vi "CMI Sync V3 Panel.vi"(8 "error in":errorcluster, 11 "session in":T2={"VISA"="", "baud rate [bd/s]"=115200, "source"=enum."Auto", "hv range"=enum."1kV", "fsrc is fixed"=FALSE, "fsrc [Hz]"=10000000.0, "freq integ [s]"=1.0, "freq filter"=5, "trig level"=enum."TTL 5V", "chn1 mode"=enum."Source divider", "chn1 level"=enum."Positive 5V", "chn2 mode"=enum."Source divider", "chn2 level"=enum."Positive 5V", "chn2 div"=1, "chn3 mode"=enum."Chn 1 Active", "chn3 level"=enum."Positive 5V", "chn1 div entry"=enum."Calculate nearest divisor from measured fx", "chn1 dev limit [%]"=1.0, "chn1 check dev"=FALSE} {"chn2 div" min=1 max=100000000 step=1; "fsrc [Hz]" format="%_8p"}) -> (0 "error out":errorcluster, 3 "session out":T2={"VISA"="", "baud rate [bd/s]"=115200, "source"=enum."Auto", "hv range"=enum."1kV", "fsrc is fixed"=FALSE, "fsrc [Hz]"=10000000.0, "freq integ [s]"=1.0, "freq filter"=5, "trig level"=enum."TTL 5V", "chn1 mode"=enum."Source divider", "chn1 level"=enum."Positive 5V", "chn2 mode"=enum."Source divider", "chn2 level"=enum."Positive 5V", "chn2 div"=1, "chn3 mode"=enum."Chn 1 Active", "chn3 level"=enum."Positive 5V", "chn1 div entry"=enum."Calculate nearest divisor from measured fx", "chn1 dev limit [%]"=1.0, "chn1 check dev"=FALSE} {"chn2 div" min=1 max=100000000 step=1; "fsrc [Hz]" format="%_8p"})   [LabVIEW 2020, in "AWG.lvlib" / "CMI Sync Unit V3.lvlib"]
doc: "Configuration panel of CMI Sync Unit V3. Sets the basic setup that is not intended to be changed after opening the device."
uses:
  CMI Sync Unit V3.lvlib
  varilib/varilib.lvlib
  varilib/SGUI Assign References Mode.ctl
  varilib/SGUI Assign Multiple Strings With Tags By Label.vi
  Configure/CMI Sync V3 Reference Clock Source.ctl
  Configure/CMI Sync V3 Channel 1 Mode.ctl
  Configure/CMI Sync V3 Channel 1 Divisor Entry Mode.ctl
  varilib/SGUI Set Single Real By Label.vi
  Configure/CMI Sync V3 HV input Range.ctl
  Configure/CMI Sync V3 Trigger Input Level.ctl
  Configure/CMI Sync V3 Channel 2 Mode.ctl
  Configure/CMI Sync V3 Channel Output Levels.ctl
  Configure/CMI Sync V3 Channel 3 Mode.ctl
  CMI Sync V3 session.ctl
panel:
  in  "chn1 freq limit":dbl=0.01 caption="Freq limit [%]" min=1e-09 max=100.0 step=0.01
  in  "chn1 check limit":bool caption="Channel 1 check deviation limit"
  in  "chn1 div entry":T1=enum."Calculate nearest divisor from measured fx" caption="Channel 1 source divider mode"
  out "err string":string caption="Error"
  out "meas freq":dbl caption="Source frequency [Hz]" format="%0_8p"
  out "idn string":string caption="Device identification"
  in  "btn check":bool
  in  "btn ok":bool caption="OK"
  in  "fsrc":dbl=10000000.0 caption="Source frequency [Hz]" format="%_8p"
  in  "fsrc fixed":bool caption="Define source freq. here:"
  in  "chn3 level":T7=enum."Positive 5V" caption="Channel 3 output levels"
  in  "chn3 mode":T9 caption="Channel 3 mode"
  in  "chn2 level":T7=enum."Positive 5V" caption="Channel 2 output levels"
  in  "chn1 level":T7=enum."Positive 5V" caption="Channel 1 output levels"
  in  "chn2 div":i32=1 caption="Channel 2 divisor" min=1 max=100000000 step=1
  in  "chn2 mode":T8 caption="Channel 2 mode"
  in  "trig level":T5=enum."TTL 5V" caption="Trigger input logic"
  in  "freq filter":i32=5 caption="Counter filtering periods"
  in  "freq integ":dbl=1.0 caption="Counter integration [s]"
  in  "chn1 mode":T6 caption="Channel 1 mode"
  in  "hv range":T4=enum."1kV" caption="HV input range"
  in  "VISA address":refnum<visa-resource-name>
  in  "source":T3 caption="Clock source"
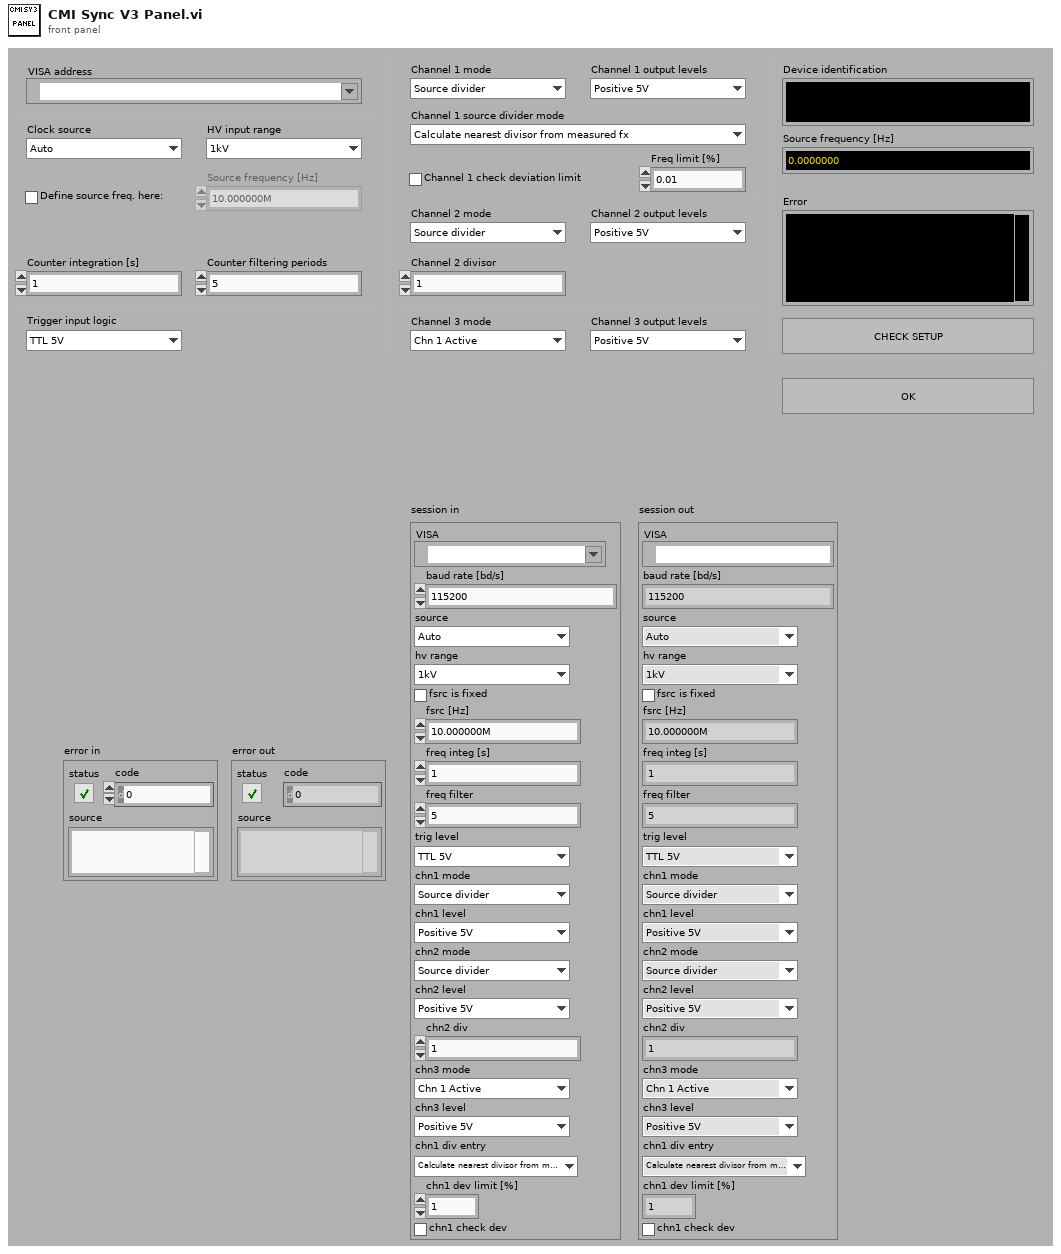
[diagram p1: front panel]
types:
  T1 = typedef "AWG.lvlib/CMI Sync Unit V3.lvlib/CMI Sync V3 Channel 1 Divisor Entry Mode.ctl" = enum16{"Set divisor directly", "Calculate nearest divisor from measured fx"}
  T2 = typedef "AWG.lvlib/CMI Sync Unit V3.lvlib/CMI Sync V3 session.ctl" = cluster{"VISA":refnum<visa-resource-name>, "baud rate [bd/s]":i32, "source":T3, "hv range":T4, "fsrc is fixed":bool, "fsrc [Hz]":dbl, "freq integ [s]":dbl, "freq filter":i32, "trig level":T5, "chn1 mode":T6, "chn1 level":T7, "chn2 mode":T8, "chn2 level":T7, "chn2 div":i32, "chn3 mode":T9, "chn3 level":T7, "chn1 div entry":T1, "chn1 dev limit [%]":dbl, "chn1 check dev":bool}
  T3 = typedef "AWG.lvlib/CMI Sync Unit V3.lvlib/CMI Sync V3 Reference Clock Source.ctl" = enum16{"Auto", "Internal", "Logic", "Sine", "HV"}
  T4 = typedef "AWG.lvlib/CMI Sync Unit V3.lvlib/CMI Sync V3 HV input Range.ctl" = enum16{"10V", "60V", "250V", "1kV"}
  T5 = typedef "AWG.lvlib/CMI Sync Unit V3.lvlib/CMI Sync V3 Trigger Input Level.ctl" = enum16{"LVCMOS 3V3", "TTL 5V"}
  T6 = typedef "AWG.lvlib/CMI Sync Unit V3.lvlib/CMI Sync V3 Channel 1 Mode.ctl" = enum16{"Source divider", "DDS absolute", "DDS ratio", "DDS ratio M/N"}
  T7 = typedef "AWG.lvlib/CMI Sync Unit V3.lvlib/CMI Sync V3 Channel Output Levels.ctl" = enum16{"Positive 3V3", "Negative 3V3", "Positive 5V", "Negative 5V"}
  T8 = typedef "AWG.lvlib/CMI Sync Unit V3.lvlib/CMI Sync V3 Channel 2 Mode.ctl" = enum16{"Source divider", "Chn 1 divide"}
  T9 = typedef "AWG.lvlib/CMI Sync Unit V3.lvlib/CMI Sync V3 Channel 3 Mode.ctl" = enum16{"Chn 1 Active", "Chn 2 Active", "Chn 1 Trigger", "Chn 2 Trigger", "Gate", "PPS", "10MHz"}
  T10 = typedef "varilib.lvlib/SGUI Assign References Mode.ctl" = enum16{"Add to stack", "Overwrite", "Release last", "Release ID"}
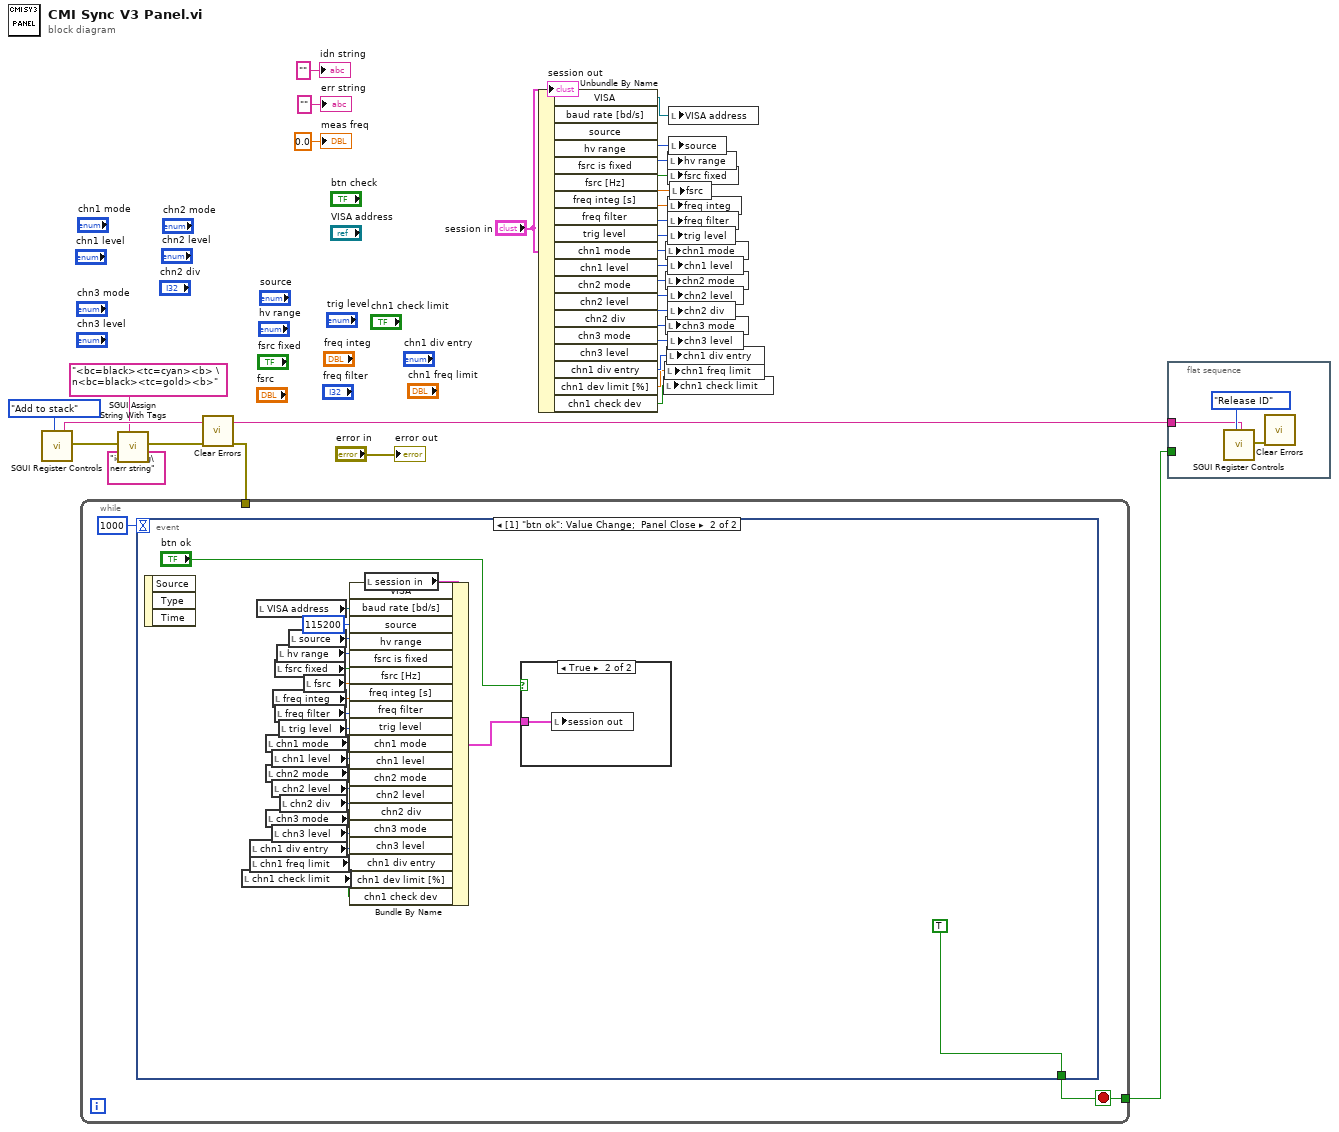
[diagram p0: block diagram]
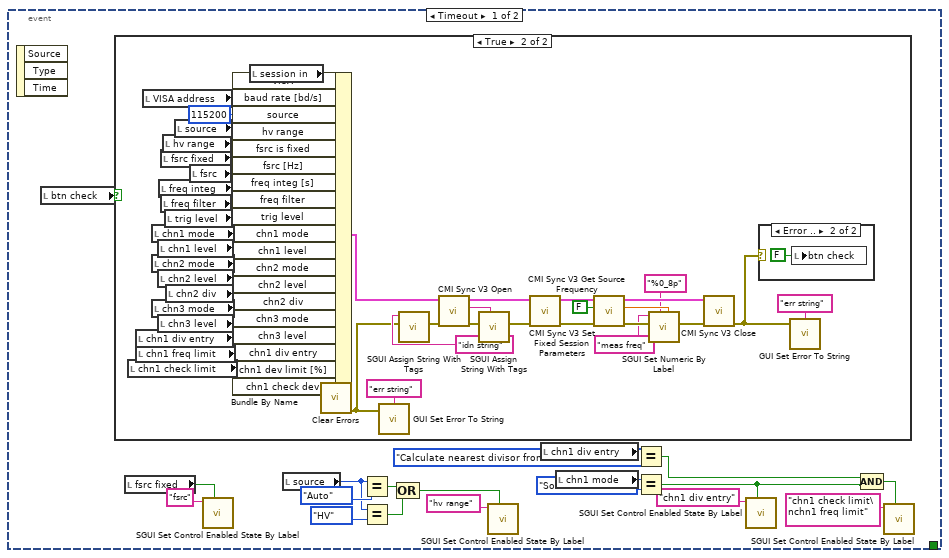
[diagram p2: hidden frame]
diagram:
  n1 = call "SGUI Register Controls.vi"("register mode (overwrite)"=SGUI_Assign_References_Mode."Add to stack") -> ("assigned ID"=w27:string, "error out"=w24:errorcluster)  [unwired: 16 in, 1 out]
  n2 = call-poly "SGUI Assign String With Tags.vi"("error in"=w24, "label(s) (empty)"="idn string\nerr string" ("control label (none)"), "string (empty)"="<bc=black><tc=cyan><b> \n<bc=black><tc=gold><b>" ("control label (none)")) -> ("error out"=w23:errorcluster)  [unwired: 7 in, 1 out]
  n3 = call <vilib>:"Clear Errors.vi"("error in (no error)"=w23) -> ("error out"=w25:errorcluster)  [unwired: 5 in, 1 out]
  n4 = while {
    tunnel: [w33] -> w26
    tunnel: w25 -> [_]
    stop <- w33 stop-if-true
    n5 = event shown="[1] \"btn ok\": Value Change;  Panel Close" {
      selector: _ -> [_ _]
      dyn-events: _ -> [_ _]
      timeout: 1000 -> [_ _]
      tunnel: [_ TRUE] -> w33
      event Timeout {
        n6 = event-data() -> ()  [unwired: 1 in, 3 out]
        n7 = local read "btn check"() -> (w52:bool)
        n8 = case shown="True" w52 {
          frame False {
          }
          frame True {
            w58 = "idn string" ("control label (none)")
            n9 = local read "chn1 check limit"() -> (w53:bool)
            n10 = local read "chn1 div entry"() -> (w55:T1)
            n11 = local read "chn1 freq limit"() -> (w54:dbl)
            n12 = local read "VISA address"() -> (w92:refnum<visa-resource-name>)
            n13 = local read "chn1 mode"() -> (w84:T6)
            n14 = local read "chn2 mode"() -> (w82:T8)
            n15 = local read "chn3 mode"() -> (w79:T9)
            n16 = local read "chn1 level"() -> (w83:T7)
            n17 = local read "chn2 level"() -> (w81:T7)
            n18 = local read "chn3 level"() -> (w78:T7)
            n19 = local read "freq integ"() -> (w87:dbl)
            n20 = local read "fsrc fixed"() -> (w89:bool)
            n21 = local read "freq filter"() -> (w86:i32)
            n22 = local read "hv range"() -> (w90:T4)
            n23 = local read "trig level"() -> (w85:T5)
            n24 = local read "chn2 div"() -> (w80:i32)
            n25 = local read "source"() -> (w91:T3)
            n26 = local read "fsrc"() -> (w88:dbl)
            n27 = local read "session in"() -> (w60:T2)
            n28 = Bundle By Name(cluster=w60, "VISA"=w92, "baud rate [bd/s]"=115200, "source"=w91, "hv range"=w90, "fsrc is fixed"=w89, "fsrc [Hz]"=w88, "freq integ [s]"=w87, "freq filter"=w86, "trig level"=w85, "chn1 mode"=w84, "chn1 level"=w83, "chn2 mode"=w82, "chn2 level"=w81, "chn2 div"=w80, "chn3 mode"=w79, "chn3 level"=w78, "chn1 div entry"=w55, "chn1 dev limit [%]"=w54, "chn1 check dev"=w53) -> (w76:T2)
            n29 = call <vilib>:"Clear Errors.vi"() -> ("error out"=w56:errorcluster)  [unwired: 6 in, 1 out]
            n30 = call "GUI Set Error To String.vi"("error in (no error)"=w56, "label(s) (status)"="err string") -> ()  [unwired: 3 in]
            n31 = call-poly "SGUI Assign String With Tags.vi"("error in"=w56, "label(s) (empty)"=w58) -> ("error out"=w59:errorcluster)  [unwired: 8 in, 1 out]
            n32 = call "CMI Sync V3 Open.vi"("error in"=w59, "session in"=w76) -> ("error out"=w69:errorcluster, "identification string"=w67:string, "session out"=w75:T2)  [unwired: 7 in]
            n33 = call-poly "SGUI Assign String With Tags.vi"("error in"=w69, "label(s) (empty)"=w58, "string (empty)"=w67) -> ("error out"=w68:errorcluster)  [unwired: 7 in, 1 out]
            n34 = call "CMI Sync V3 Set Fixed Session Parameters.vi"("error in"=w68, "session in"=w75) -> ("error out"=w74:errorcluster, "session out"=w73:T2)  [unwired: 8 in]
            n35 = call "CMI Sync V3 Get Source Frequency.vi"("error in"=w74, "Wait for update before? (false)"=FALSE, "session in"=w73) -> ("error out"=w66:errorcluster, "source frequency [Hz]"=w64:dbl, "session out"=w72:T2)  [unwired: 6 in]
            n36 = call-poly "SGUI Set Numeric By Label.vi"("error in"=w66, "label (empty)"="meas freq", "format (empty)"="%0_8p", "value (none)"=w64) -> ("error out"=w65:errorcluster)  [unwired: 6 in, 1 out]
            n37 = call "CMI Sync V3 Close.vi"("error in"=w65, "session in"=w72) -> ("error out"=w70:errorcluster)  [unwired: 8 in, 1 out]
            n38 = case shown="Error .." w70 {
              frame No Error {
              }
              frame Error {
                n39 = local write "btn check"(FALSE ("btn check")) -> ()
              }
            }
            n40 = call "GUI Set Error To String.vi"("error in (no error)"=w70, "label(s) (status)"="err string") -> ()  [unwired: 3 in]
          }
        }
        n41 = local read "fsrc fixed"() -> (w51:bool)
        n42 = call "SGUI Set Control Enabled State By Label.vi"("labels (empty)"="fsrc", "Enabled? (False)"=w51) -> ()  [unwired: 8 in, 2 out]
        n43 = local read "source"() -> (w47:T3)
        n44 = Equal?(x=w47, y=CMI_Sync_V3_Reference_Clock_Source."Auto") -> (x = y?=w45:bool)
        n45 = Equal?(x=w47, y=CMI_Sync_V3_Reference_Clock_Source."HV") -> (x = y?=w44:bool)
        n46 = Compound Arithmetic op=OR(w45, w44) -> (w43:bool)
        n47 = call "SGUI Set Control Enabled State By Label.vi"("labels (empty)"="hv range", "Enabled? (False)"=w43) -> ()  [unwired: 8 in, 2 out]
        n48 = local read "chn1 div entry"() -> (w38:T1)
        n49 = local read "chn1 mode"() -> (w42:T6)
        n50 = Equal?(x=w38, y=CMI_Sync_V3_Channel_1_Divisor_Entry_Mode."Calculate nearest divisor from measured fx") -> (x = y?=w35:bool)
        n51 = Equal?(x=w42, y=CMI_Sync_V3_Channel_1_Mode."Source divider") -> (x = y?=w36:bool)
        n52 = call "SGUI Set Control Enabled State By Label.vi"("labels (empty)"="chn1 div entry", "Enabled? (False)"=w36) -> ()  [unwired: 8 in, 2 out]
        n53 = Compound Arithmetic op=AND(w35, w36) -> (w34:bool)
        n54 = call "SGUI Set Control Enabled State By Label.vi"("labels (empty)"="chn1 check limit\nchn1 freq limit", "Enabled? (False)"=w34) -> ()  [unwired: 8 in, 2 out]
      }
      event "btn ok": Value Change; Panel Close {
        n55 = event-data() -> ()  [unwired: 1 in, 3 out]
        n56 = local read "chn1 check limit"() -> (w94:bool)
        n57 = local read "chn1 div entry"() -> (w96:T1)
        n58 = local read "chn1 freq limit"() -> (w95:dbl)
        n59 = local read "VISA address"() -> (w116:refnum<visa-resource-name>)
        n60 = local read "chn1 mode"() -> (w107:T6)
        n61 = local read "chn2 mode"() -> (w105:T8)
        n62 = local read "chn3 mode"() -> (w102:T9)
        n63 = local read "chn1 level"() -> (w106:T7)
        n64 = local read "chn2 level"() -> (w104:T7)
        n65 = local read "chn3 level"() -> (w101:T7)
        n66 = local read "freq integ"() -> (w110:dbl)
        n67 = local read "fsrc fixed"() -> (w112:bool)
        n68 = local read "freq filter"() -> (w109:i32)
        n69 = local read "hv range"() -> (w113:T4)
        n70 = local read "trig level"() -> (w108:T5)
        n71 = local read "chn2 div"() -> (w103:i32)
        n72 = local read "source"() -> (w114:T3)
        n73 = local read "fsrc"() -> (w111:dbl)
        n74 = local read "session in"() -> (w99:T2)
        n75 = Bundle By Name(cluster=w99, "VISA"=w116, "baud rate [bd/s]"=115200, "source"=w114, "hv range"=w113, "fsrc is fixed"=w112, "fsrc [Hz]"=w111, "freq integ [s]"=w110, "freq filter"=w109, "trig level"=w108, "chn1 mode"=w107, "chn1 level"=w106, "chn2 mode"=w105, "chn2 level"=w104, "chn2 div"=w103, "chn3 mode"=w102, "chn3 level"=w101, "chn1 div entry"=w96, "chn1 dev limit [%]"=w95, "chn1 check dev"=w94) -> (w98:T2)
        n76 = case shown="True" "btn ok" {
          tunnel: w98 -> [_ w117]
          frame False {
          }
          frame True {
            n77 = local write "session out"(w117) -> ()
          }
        }
      }
    }
  }
  n78 = Unbundle By Name("session in") -> ("VISA"=w19:refnum<visa-resource-name>, "source"=w18:T3, "hv range"=w17:T4, "fsrc is fixed"=w16:bool, "fsrc [Hz]"=w15:dbl, "freq integ [s]"=w14:dbl, "freq filter"=w13:i32, "trig level"=w12:T5, "chn1 mode"=w11:T6, "chn1 level"=w10:T7, "chn2 mode"=w9:T8, "chn2 level"=w8:T7, "chn2 div"=w7:i32, "chn3 mode"=w6:T9, "chn3 level"=w5:T7, "chn1 div entry"=w3:T1, "chn1 dev limit [%]"=w2:dbl, "chn1 check dev"=w1:bool)  [unwired: 1 out]
  n79 = local write "chn1 check limit"(w1) -> ()
  n80 = local write "chn1 freq limit"(w2) -> ()
  n81 = local write "chn1 mode"(w11) -> ()
  n82 = local write "chn2 mode"(w9) -> ()
  n83 = local write "chn3 mode"(w6) -> ()
  n84 = local write "chn1 div entry"(w3) -> ()
  n85 = local write "hv range"(w17) -> ()
  n86 = local write "fsrc fixed"(w16) -> ()
  n87 = local write "freq integ"(w14) -> ()
  n88 = local write "freq filter"(w13) -> ()
  n89 = local write "trig level"(w12) -> ()
  n90 = local write "chn1 level"(w10) -> ()
  n91 = local write "chn2 level"(w8) -> ()
  n92 = local write "chn2 div"(w7) -> ()
  n93 = local write "chn3 level"(w5) -> ()
  n94 = local write "VISA address"(w19) -> ()
  n95 = local write "source"(w18) -> ()
  n96 = local write "fsrc"(w15) -> ()
  n97 = flat-sequence {
    tunnel: w27 -> [w119]
    tunnel: w26 -> [_]
    frame #0 {
      n98 = call "SGUI Register Controls.vi"("register mode (overwrite)"=SGUI_Assign_References_Mode."Release ID", "controls ID (empty)"=w119) -> ("error out"=w118:errorcluster)  [unwired: 15 in, 2 out]
      n99 = call <vilib>:"Clear Errors.vi"("error in (no error)"=w118) -> ()  [unwired: 5 in, 2 out]
    }
  }
  "idn string" <- "" ("idn string")
  "meas freq" <- 0.0 ("meas freq")
  "err string" <- "" ("err string")
  "session out" <- "session in"
  "error out" <- "error in"
